vi "SendStreamData.vi"(8 "Error In":errorcluster, 9 "Timeout (ms)":i32, 10 "ServerStreamData":T1, 11 "Connection In":T6={"UDP Connection ID"=refnum, "TCP Connection ID"=refnum, "Remote UDP Port"=61557, "Remote IP"=0}) -> (0 "Error Out":errorcluster, 3 "Connection Out":T6={"UDP Connection ID"=refnum, "TCP Connection ID"=refnum, "Remote UDP Port"=61557, "Remote IP"=0}, 4 "stop?":bool)   [LabVIEW 2017, in "Game.lvlib" / "GameComms.lvlib"]
uses:
  GameComms.lvlib
  TypeDefs/Connection.ctl
  TypeDefs/ServerStreamData.ctl
  TypeDefs/HandPosition.ctl
  TypeDefs/ElbowPosition.ctl
  TypeDefs/ShoulderPosition.ctl
  TypeDefs/UserInput.ctl
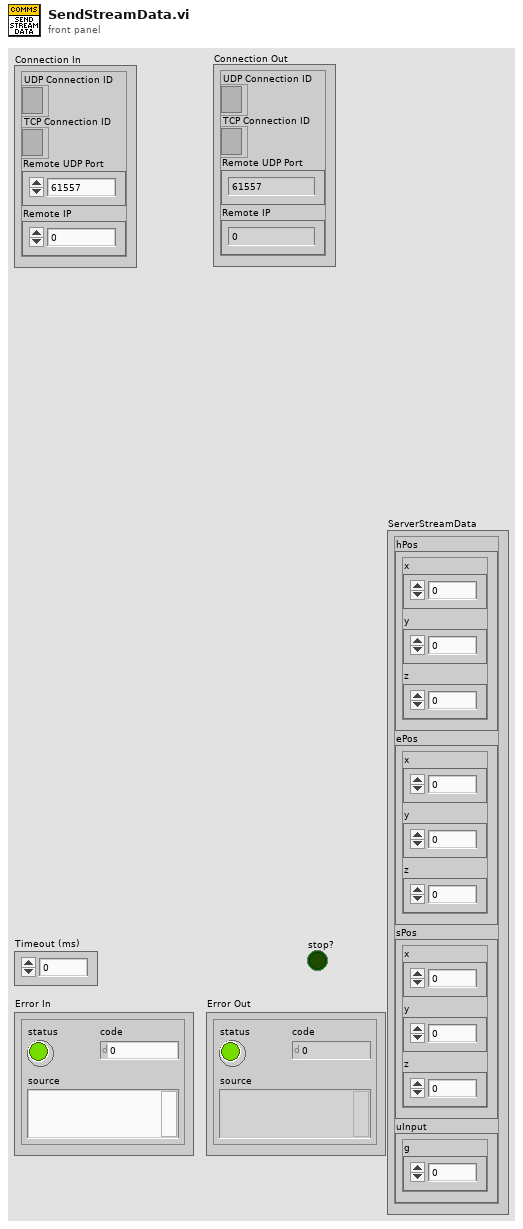
[diagram p1: front panel]
types:
  T1 = typedef "Game.lvlib/GameComms.lvlib/ServerStreamData.ctl" = cluster{"hPos":T2, "ePos":T3, "sPos":T4, "uInput":T5}
  T2 = typedef "Game.lvlib/GameComms.lvlib/HandPosition.ctl" = cluster{"x":dbl, "y":dbl, "z":dbl}
  T3 = typedef "Game.lvlib/GameComms.lvlib/ElbowPosition.ctl" = cluster{"x":dbl, "y":dbl, "z":dbl}
  T4 = typedef "Game.lvlib/GameComms.lvlib/ShoulderPosition.ctl" = cluster{"x":dbl, "y":dbl, "z":dbl}
  T5 = typedef "Game.lvlib/GameComms.lvlib/UserInput.ctl" = cluster{"g":dbl}
  T6 = typedef "Game.lvlib/GameComms.lvlib/Connection.ctl" = cluster{"UDP Connection ID":refnum<k16>, "TCP Connection ID":refnum<k5>, "Remote UDP Port":u16, "Remote IP":u32}
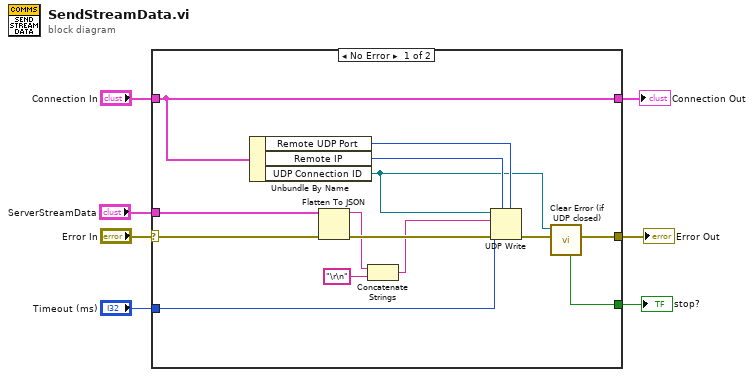
[diagram p0: block diagram]
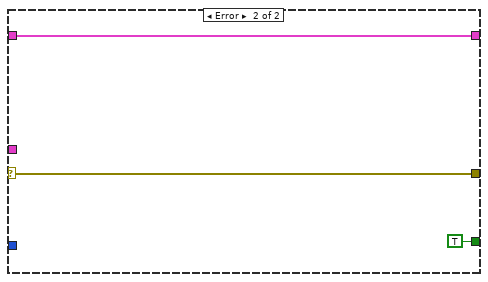
[diagram p2: hidden frame]
diagram:
  n1 = case shown="No Error" "Error In" {
    selector: "Error In" -> [w16 w24]
    tunnel: [w9 w24] -> w6
    tunnel: "Connection In" -> [w13 w23]
    tunnel: "ServerStreamData" -> [w17 _]
    tunnel: [w13 w23] -> w4
    tunnel: "Timeout (ms)" -> [w12 _]
    tunnel: [w8 TRUE ("stop?")] -> w1
    frame No Error {
      n2 = Unbundle By Name(w13) -> ("Remote UDP Port"=w14:u16, "Remote IP"=w15:u32, "UDP Connection ID"=w11:refnum<k16>)
      n3 = Flatten To JSON(anything=w17, error in (no error)=w16) -> (JSON string=w19:string, 11:w21:errorcluster)  [unwired: 1 in]
      n4 = Concatenate Strings(w19, "\r\n" ("string")) -> (w18:string)
      n5 = UDP Write(address=w15, port or service name=w14, connection ID=w11, data in=w18, 8:w21, 9:w12) -> (error out=w10:errorcluster)  [unwired: 1 out]
      n6 = call "Clear Error (if UDP closed).vi"("error in"=w10, "udp refnum"=w11) -> ("error out"=w9:errorcluster, "stop?"=w8:bool)  [unwired: 8 in]
    }
    frame Error {
    }
  }
  "Error Out" <- w6
  "Connection Out" <- w4
  "stop?" <- w1
